vi "GoToAngleVSS.vi"(10 "orientation":dbl format="%#_13g", 11 "dest_orientation":dbl) -> (3 "v_ang":dbl)   [LabVIEW 2018]
panel:
  in  "Limits":cluster{"output high":dbl, "output low":dbl}={"output high"=100.0, "output low"=-100.0}
  in  "PID gains in":T1={"proportional gain (Kc)"=2.3, "integral time (Ti, min)"=0.0, "derivative time (Td, min)"=2.5}
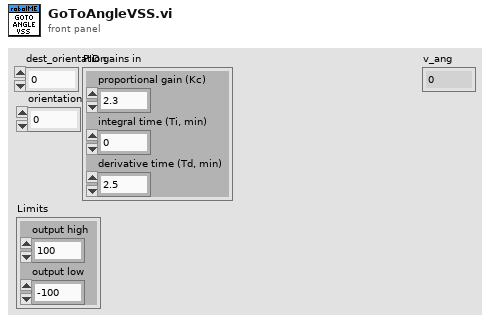
[diagram p1: front panel]
types:
  T1 = cluster{"proportional gain (Kc)":dbl, "integral time (Ti, min)":dbl, "derivative time (Td, min)":dbl}
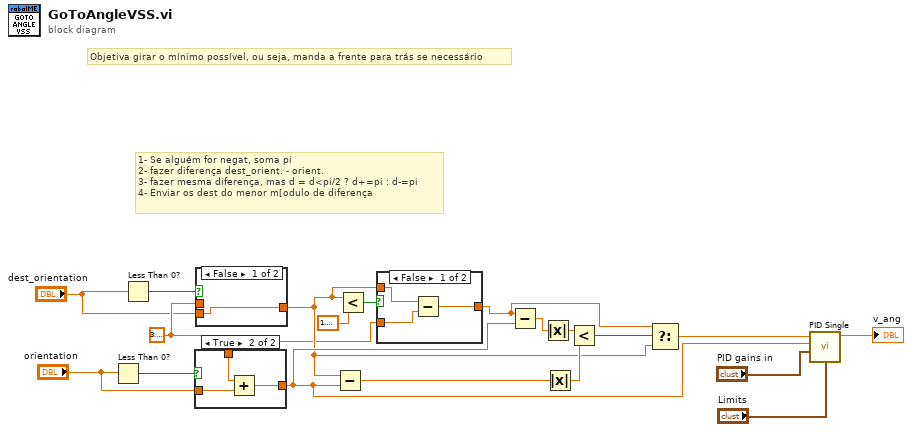
[diagram p0: block diagram]
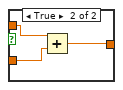
[diagram p2: hidden frame]
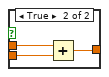
[diagram p4: hidden frame]
diagram:
  w2 = 3.141592653589793
  # "Objetiva girar o mínimo possível, ou seja, manda a frente para trás se necessário"
  # "1- Se alguém for negat, soma pi\n2- fazer diferença dest_orient. - orient.\n3- fazer mesma diferença, mas d = d<pi/2 ? d+=pi : d-=pi\n4- Enviar os dest do menor m[odulo de diferença"
  n1 = Less Than 0?(x="orientation") -> (x < 0?=w16:bool)
  n2 = Less Than 0?(x="dest_orientation") -> (x < 0?=w15:bool)
  n3 = case shown="True" w16 {
    tunnel: "orientation" -> [w20 w23]
    tunnel: [w20 w22] -> w6
    tunnel: w2 -> [_ w21]
    frame False {
    }
    frame True {
      n4 = Add(x=w21, y=w23) -> (x+y=w22:dbl)
    }
  }
  n5 = case shown="False" w15 {
    tunnel: "dest_orientation" -> [w24 w27]
    tunnel: [w24 w26] -> w4
    tunnel: w2 -> [_ w25]
    frame False {
    }
    frame True {
      n6 = Add(x=w25, y=w27) -> (x+y=w26:dbl)
    }
  }
  n7 = Subtract(x=w4, y=w6) -> (x-y=w8:dbl)
  n8 = Less?(x=w4, y=1.5707963267948966) -> (x < y?=w13:bool)
  n9 = case shown="False" w13 {
    tunnel: w2 -> [w29 w33]
    tunnel: w4 -> [w30 w32]
    tunnel: [w28 w31] -> w5
    frame False {
      n10 = Subtract(x=w30, y=w29) -> (x-y=w28:dbl)
    }
    frame True {
      n11 = Add(x=w32, y=w33) -> (x+y=w31:dbl)
    }
  }
  n12 = Subtract(x=w5, y=w6) -> (x-y=w11:dbl)
  n13 = Absolute Value(x=w11) -> (abs(x)=w10:dbl)
  n14 = Absolute Value(x=w8) -> (abs(x)=w9:dbl)
  n15 = Less?(x=w10, y=w9) -> (x < y?=w7:bool)
  n16 = Select(t=w5, s=w7, f=w4) -> (s? t:f=w3:dbl)
  n17 = call "PID Single.vi"("Limits"="Limits", "PID gains in"="PID gains in", "Variable"=w6, "Setpoint"=w3) -> ("Out"=→"v_ang":dbl)  [unwired: 7 in]
